vi "Preiniger Bartosz praca inżynierska.vi"() -> ()   [LabVIEW 2021]
uses:
  <vilib>/sound2/lvsound2.llb/Sound Data Format.ctl
  <vilib>/sound2/lvsound2.llb/Sampling Mode.ctl
  <vilib>/sound2/lvsound2.llb/Sound Output Set Volume (Single).vi
  <vilib>/sound2/lvsound2.llb/Sound Output Write (DBL Single).vi
  <vilib>/measure/NI_MABase.lvlib
  user32.dll
panel:
  in  "Tab Control":enum32{"Page 1", "Page 2"}(tab)
  in  "Częstotliwość":dbl(knob)=10.0 min=10.0 max=20000.0 step=1.0 scale=10.0..20000.0
  out "Boolean":bool
  in  "on/off":bool
  out "Wykres generowanego przebiegu":waveform(dbl)(graph)
  in  "Procent napięcia maksymalnego":dbl(knob) min=0.0 max=100.0 step=1.0 scale=0.0..100.0
  in  "Rodzaj przebiegu":T1(ring)
  in  "Wyłącz":bool
  # "Generator sygnałów testowych"
  # "%"
  # "Hz"
  # "ON"
  # "Output"
  # "OFF"
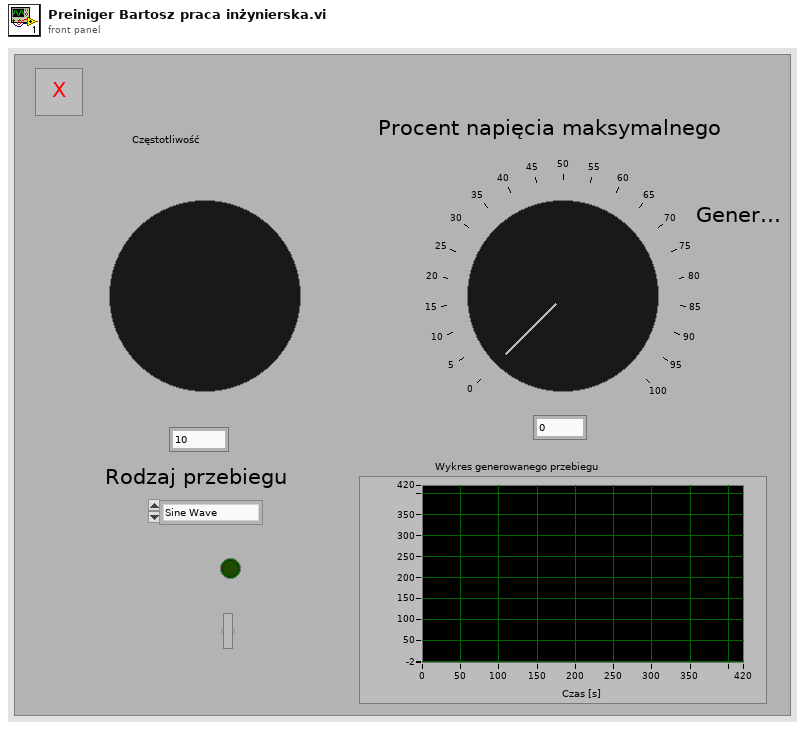
[diagram p1: front panel]
types:
  T1 = enum16{"Sine Wave", "Triangle Wave", "Square Wave", "Sawtooth Wave"}
  T2 = typedef "Sampling Mode.ctl" = i32
  T3 = typedef "Sound Data Format.ctl" = cluster{"sample rate (S/s)":dbl, "number of channels":i32, "bits per sample":i32}
  T4 = typedef "Sound Output Task ID.ctl" = u32
  T5 = cluster{"sample rate (S/s)":dbl, "number of samples/ch":i32}
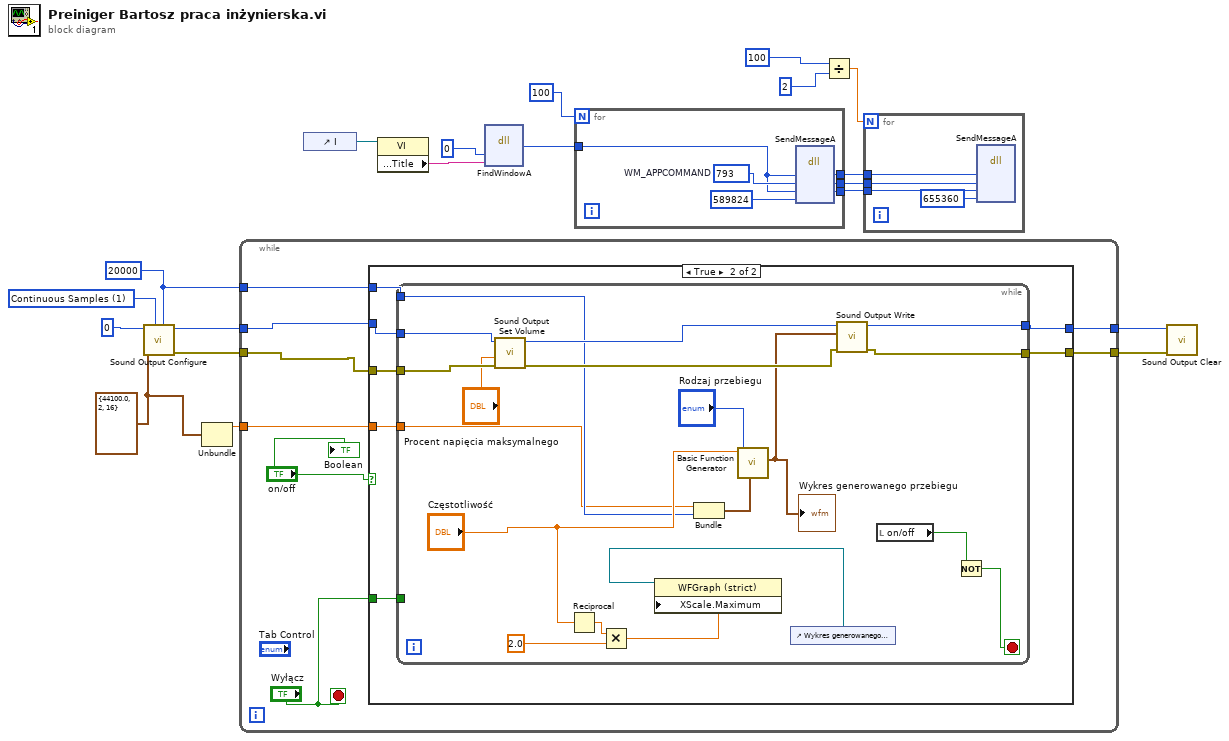
[diagram p0: block diagram]
diagram:
  w13 = 20000 ("number of samples/ch")
  w15 = T2 1 items=["Finite Samples", "Continuous Samples"] ("sample mode")
  w14 = T3 {"sample rate (S/s)"=44100.0, "number of channels"=2, "bits per sample"=16} ("sound format")
  n1 = call <vilib>:"Sound Output Configure.vi"("number of samples/ch"=w13, "sample mode"=w15, "sound format"=w14, "device ID"=u32 0) -> ("error out"=w17:errorcluster, "task ID"=w19:T4)  [unwired: 6 in]
  n2 = Unbundle(w14) -> ("sample rate (S/s)"=w12:dbl)  [unwired: 2 out]
  n3 = while {
    tunnel: w19 -> [w28]
    tunnel: [w25] -> w18
    tunnel: w17 -> [w27]
    tunnel: [w26] -> w16
    tunnel: w13 -> [w24]
    tunnel: w12 -> [w23]
    stop <- "Wyłącz" stop-if-true
    n4 = case shown="True" "on/off" {
      tunnel: w28 -> [w30 w37]
      tunnel: w27 -> [w29 w36]
      tunnel: [w29 w35] -> w26
      tunnel: [w30 w34] -> w25
      tunnel: w24 -> [_ w33]
      tunnel: w23 -> [_ w32]
      tunnel: "Wyłącz" -> [_ w31]
      frame False {
      }
      frame True {
        n5 = while {
          tunnel: w36 -> [w56]
          tunnel: [w46] -> w35
          tunnel: w37 -> [w45]
          tunnel: [w44] -> w34
          tunnel: w33 -> [w41]
          tunnel: w32 -> [w40]
          tunnel: w31 -> [_]
          stop <- w38 stop-if-true
          n6 = call-poly <vilib>:"Sound Output Set Volume.vi"("error in (no error)"=w56, "volume"="Procent napięcia maksymalnego", "task ID"=w45) -> ("error out"=w55:errorcluster, "task ID out"=w54:T4)  [unwired: 7 in]
          n7 = Reciprocal(x="Częstotliwość") -> (1/x=w49:dbl)
          n8 = Multiply(x=w49, y=2.0) -> (x*y=w50:dbl)
          n9 = Bundle("sample rate (S/s)"=w40, "number of samples/ch"=w41) -> (w42:T5)  [unwired: 1 in]
          n10 = call <vilib>:"Basic Function Generator.vi"("sampling info"=w42, "signal type"="Rodzaj przebiegu", "frequency"="Częstotliwość") -> ("signal out"=w47:waveform(dbl))  [unwired: 6 in, 2 out]
          "Wykres generowanego przebiegu" <- w47
          n11 = control-ref of="Wykres generowanego przebiegu"() -> (w51:refnum<vi>)
          n12 = property on="Property Node" class="WFGraph (strict)"(reference=w51, "XScale.Maximum"=w50) -> ()  [unwired: 1 in, 2 out]
          n13 = call-poly <vilib>:"Sound Output Write.vi"("error in (no error)"=w55, "data"=w47, "task ID"=w54) -> ("error out"=w46:errorcluster, "task ID out"=w44:T4)  [unwired: 7 in]
          n14 = local read "on/off"() -> (w39:bool)
          n15 = Not(x=w39) -> (.not. x?=w38:bool)
        }
      }
    }
    "Boolean" <- "on/off"
  }
  n16 = control-ref of="I"() -> (w10:refnum<vi>)
  n17 = property class="VI"(reference=w10) -> ("Front Panel.Title"=w9:string)  [unwired: 1 in, 2 out]
  n18 = dll-call lib="user32.dll" fn="FindWindowA"("lpszClassName"=0, "lpszWindowName"=w9) -> ("hWnd"=w8:u32)  [unwired: 5 in, 2 out]
  n19 = for {
    N: 100 -> [_]
    tunnel: w8 -> [w60]
    tunnel: [w59] -> w7
    tunnel: [w58] -> w6
    tunnel: [w57] -> w5
    w62 = u32 793  # WM_APPCOMMAND
    n20 = dll-call lib="user32.dll" fn="SendMessageA"("hWnd"=w60, "Msg"=w62, "wParam"=w60, "lParam"=589824) -> ("hWnd"=w58:u32, "Msg"=w57:u32, "wParam"=w59:u32)  [unwired: 5 in, 2 out]
  }
  n21 = Divide(x=100, y=2) -> (x/y=w2:dbl)
  n22 = for {
    N: w2 -> [_]
    tunnel: w7 -> [w65]
    tunnel: w6 -> [w64]
    tunnel: w5 -> [w63]
    n23 = dll-call lib="user32.dll" fn="SendMessageA"("hWnd"=w64, "Msg"=w63, "wParam"=w65, "lParam"=655360) -> ()  [unwired: 8 in, 2 out]
  }
  n24 = call <vilib>:"Sound Output Clear.vi"("error in (no error)"=w16, "task ID"=w18) -> ()  [unwired: 9 in, 1 out]
